vi "UHR-Fleezers Control (host) - 11.1.vi"() -> ()   [LabVIEW 2012] (continued)
            n680 = call "move to saved stage position.vi"("error in"=w1090, "Stage VISA resource name in"=w1091, "Position"="Stage Position To Establish FB", "Saved Stage Positions"=w1093) -> ("error out"=w1089:errorcluster)  [unwired: 1 out]
            n681 = local write "Stage Control Serial Error"(w1089) -> ()
          }
          frame #2 {
            n682 = call <vilib>:"Beep.vi"() -> ()  [unwired: 3 in, 9 out]
            n683 = Multiply(x="Wait (s)", y=u32 1000 ("milliseconds to wait")) -> (x*y=w1099:u32)
            n684 = property on="Trap Delta (MHz)" class="DigNum (strict)"("Val(Sgnl)"="Starting \nTrap Delta (MHz)") -> ()  [unwired: 2 in, 2 out]
            n685 = local write "Stage Moving"(FALSE ("Stage Moving")) -> ()
            n686 = Wait (ms)(milliseconds to wait=w1099) -> ()  [unwired: 1 out]
            n687 = property on="Tab Control 2" class="TabCtl (strict)"("Val(Sgnl)"=T6."Feedback on Trap Position" ("Value (Signaling)")) -> ()  [unwired: 2 in, 2 out]
            n688 = property on="Tab Control" class="TabCtl (strict)"("Val(Sgnl)"=T4."Trap Control (RF)" ("Value (Signaling)")) -> ()  [unwired: 2 in, 2 out]
          }
          frame #3 {
            n689 = property on="Set Reading to\nSetpoint" class="Bool (strict)"("Val(Sgnl)"=TRUE ("Value (Signaling)")) -> ()  [unwired: 2 in, 2 out]
            n690 = Wait (ms)(milliseconds to wait=u32 500) -> ()  [unwired: 1 out]
          }
          frame #4 {
            n691 = property on="Trap Pos. FB ON" class="Bool (strict)"("Val(Sgnl)"=TRUE ("Value (Signaling)")) -> ()  [unwired: 2 in, 2 out]
            n692 = Wait (ms)(milliseconds to wait=u32 250) -> ()  [unwired: 1 out]
          }
          frame #5 {
            n693 = case shown="False" "Trap Trig Fl." {
              frame False {
                n694 = case shown="True" "Green ON after FB ON?" {
                  selector: "Green ON after FB ON?" -> [_ w1115]
                  frame False {
                  }
                  frame True {
                    n695 = property on="Green Laser ON/Interlacing" class="Bool (strict)"("Val(Sgnl)"=w1115) -> ()  [unwired: 2 in, 2 out]
                  }
                }
              }
              frame True {
              }
            }
            n696 = case shown="True" "Remove Action Offset" {
              tunnel: TRUE ("Value (Signaling)") -> [w1112 w1113]
              frame False {
                n697 = property on="Remove Unwinding Offset" class="Bool (strict)"("Val(Sgnl)"=w1112) -> ()  [unwired: 2 in, 2 out]
              }
              frame True {
                n698 = property on="Remove Action Offset" class="Bool (strict)"("Val(Sgnl)"=w1113) -> ()  [unwired: 2 in, 2 out]
              }
            }
            n699 = Wait (ms)(milliseconds to wait=u32 250) -> ()  [unwired: 1 out]
          }
          frame #6 {
            n700 = property on="Start Saving" class="Bool (strict)"("Val(Sgnl)"=TRUE ("Value (Signaling)")) -> ()  [unwired: 2 in, 2 out]
            n701 = Wait (ms)(milliseconds to wait=u32 5000) -> ()  [unwired: 1 out]
          }
          frame #7 {
            w1119 = TRUE ("Value (Signaling)")
            n702 = property on="Rem fb disp offset" class="Bool (strict)"("Val(Sgnl)"=w1119) -> ()  [unwired: 2 in, 2 out]
            n703 = property on="Remove Offset" class="Bool (strict)"("Val(Sgnl)"=w1119) -> ()  [unwired: 2 in, 2 out]
            n704 = Wait (ms)(milliseconds to wait=u32 100) -> ()  [unwired: 1 out]
          }
          frame #8 {
            n705 = case shown="True" w1122 {
              frame False {
              }
              frame True {
                n706 = local write "Trap Trig. Fl."(TRUE ("Value (Signaling)")) -> ()
              }
            }
          }
          frame #9 {
            n707 = case shown="True" "Start dipping after?" {
              frame False {
              }
              frame True {
                n708 = flat-sequence {
                  frame #0 {
                    n709 = Multiply(x="Delay before dipping (s)", y=1000.0) -> (x*y=w1126:dbl)
                    n710 = Wait (ms)(milliseconds to wait=w1126) -> ()  [unwired: 1 out]
                  }
                  frame #1 {
                    n711 = property on="Dip for Protein" class="Bool (strict)"("Val(Sgnl)"=TRUE ("Value (Signaling)")) -> ()  [unwired: 2 in, 2 out]
                    n712 = local write "Scripts"(T1."Dipping" ("Scripts")) -> ()
                  }
                }
              }
            }
          }
        }
      }
      event "Fixed Traps Data\nScript": Value Change {
        n713 = event-data() -> ()  [unwired: 1 in, 5 out]
        n714 = flat-sequence {
          frame #0 {
            n715 = case shown="True" "Green ON" {
              frame False {
              }
              frame True {
                n716 = property on="Green Laser ON/Interlacing" class="Bool (strict)"("Val(Sgnl)"=TRUE) -> ()  [unwired: 2 in, 2 out]
              }
            }
            n717 = local write "Offset (nm)"(0.0 ("Offset (nm)")) -> ()
            n718 = property on="Sample Channel\nFlow" class="Bool (strict)"("Val(Sgnl)"=FALSE ("Value (Signaling)")) -> ()  [unwired: 2 in, 2 out]
            n719 = property on="Trap Delta (MHz)" class="DigNum (strict)"("Val(Sgnl)"="Fixed Traps Trap Delta (MHz)") -> ()  [unwired: 2 in, 2 out]
          }
          frame #1 {
            n720 = Wait (ms)(milliseconds to wait=u32 1000) -> ()  [unwired: 1 out]
          }
          frame #2 {
            n721 = local write "Start Saving"(TRUE ("Start Saving")) -> ()
          }
          frame #3 {
            n722 = local read "Bead Sep. Int. Time (s)"() -> (w1137:dbl)
            n723 = Multiply(x=w1137, y=1000.0) -> (x*y=w1139:dbl)
            n724 = Wait (ms)(milliseconds to wait=w1139) -> ()  [unwired: 1 out]
          }
          frame #4 {
            n725 = property on="Remove Offset" class="Bool (strict)"("Val(Sgnl)"=TRUE ("Value (Signaling)")) -> ()  [unwired: 2 in, 2 out]
          }
          frame #5 {
            n726 = property on="Dip for Protein" class="Bool (strict)"("Val(Sgnl)"="Start dipping after?") -> ()  [unwired: 2 in, 2 out]
          }
        }
      }
      event "Got DNA bead": Value Change {
        n727 = event-data() -> ()  [unwired: 1 in, 5 out]
        n728 = flat-sequence {
          frame #0 {
            n729 = local read "Daq spot flow on"() -> (w1144:bool)
            n730 = case shown="True" w1144 {
              frame False {
              }
              frame True {
                n731 = property on="Sample Channel\nFlow" class="Bool (strict)"("Val(Sgnl)"=TRUE ("Value (Signaling)")) -> ()  [unwired: 2 in, 2 out]
              }
            }
            n732 = property on="Got DNA bead" class="Bool"("Key Focus"=FALSE) -> ()  [unwired: 2 in, 2 out]
          }
          frame #1 {
            n733 = property on="Inject Pump 1" class="Bool (strict)"("Val(Sgnl)"=FALSE ("Value (Signaling)")) -> ()  [unwired: 2 in, 2 out]
          }
          frame #2 {
            n734 = property on="Cal/Data Acq. Spot" class="Bool (strict)"("Val(Sgnl)"=TRUE ("Value (Signaling)")) -> ()  [unwired: 2 in, 2 out]
          }
        }
      }
      event "Take Stepping Data": Value Change {
        n735 = event-data() -> ()  [unwired: 1 in, 5 out]
        n736 = local read "Save ave N"() -> (w1156:dbl)
        n737 = flat-sequence {
          tunnel: w1156 -> [w1158]
          tunnel: [w1158] -> w1151
          tunnel: [w1160] -> w1152
          tunnel: w1151 -> [w1160]
          tunnel: [w1162] -> w1153
          tunnel: w1152 -> [w1162]
          tunnel: [w1165] -> w1154
          tunnel: w1153 -> [w1165]
          tunnel: [w1167] -> w1155
          tunnel: w1154 -> [w1167]
          tunnel: [w1169] -> w1149
          tunnel: w1155 -> [w1169]
          tunnel: w1149 -> [w1172]
          tunnel: [w1172] -> w1148
          tunnel: w1148 -> [w1173]
          tunnel: [w1173] -> w1150
          tunnel: w1150 -> [w1179]
          frame #0 {
            n738 = property on="Save ave N" class="DigNum (strict)"("Val(Sgnl)"="Save ave factor") -> ()  [unwired: 2 in, 2 out]
          }
          frame #1 {
            n739 = Wait (ms)(milliseconds to wait=u32 100) -> ()  [unwired: 1 out]
          }
          frame #2 {
            n740 = local read "Offset 2 Start (MHz)"() -> (w1164:dbl)
            n741 = property on="Saved AOD Raster Scan Parameter Sets" class="Arr (strict)"("Index Values"=u32[] [2]) -> ()  [unwired: 2 in, 2 out]
            n742 = property on="Trap Delta (MHz)" class="DigNum (strict)"("Val(Sgnl)"=w1164) -> ()  [unwired: 2 in, 2 out]
          }
          frame #3 {
            n743 = property on="Load parameters" class="Bool (strict)"("Val(Sgnl)"=TRUE ("Value (Signaling)")) -> ()  [unwired: 2 in, 2 out]
          }
          frame #4 {
            n744 = Wait (ms)(milliseconds to wait=u32 100) -> ()  [unwired: 1 out]
          }
          frame #5 {
            n745 = property on="Trap Raster Scan" class="Bool (strict)"("Val(Sgnl)"=TRUE ("Value (Signaling)")) -> ()  [unwired: 2 in, 2 out]
          }
          frame #6 {
            n746 = Wait (ms)(milliseconds to wait=u32 1000) -> ()  [unwired: 1 out]
          }
          frame #7 {
            n747 = while {
              stop <- w1176 stop-if-true
              n748 = local read "Raster Scanning..."() -> (w1178:bool)
              n749 = local read "Saving..."() -> (w1177:bool)
              n750 = Not(x=w1177) -> (.not. x?=w1174:bool)
              n751 = Not(x=w1178) -> (.not. x?=w1175:bool)
              n752 = And(x=w1175, y=w1174) -> (x .and. y?=w1176:bool)
            }
          }
          frame #8 {
            n753 = property on="Save ave N" class="DigNum (strict)"("Val(Sgnl)"=w1179) -> ()  [unwired: 2 in, 2 out]
          }
        }
      }
      event "Step Size (nm)": Value Change {
        n754 = event-data() -> ()  [unwired: 1 in, 5 out]
        n755 = flat-sequence {
          frame #0 {
            n756 = property on="Saved AOD Raster Scan Parameter Sets" class="Arr (strict)"("Index Values"=u32[] [1]) -> ()  [unwired: 2 in, 2 out]
          }
          frame #1 {
            n757 = Multiply(x="N Steps", y="Step Size (nm)") -> (x*y=w1181:dbl)
            n758 = property on="Scan Speed AOD (nm/s) 2" class="DigNum (strict)"("Value"="Step Size (nm)") -> ()  [unwired: 2 in, 2 out]
            n759 = property on="Step Size AOD (nm) 2" class="DigNum (strict)"("Value"="Step Size (nm)") -> ()  [unwired: 2 in, 2 out]
            n760 = property on="Scan Range AOD (nm) 2" class="DigNum (strict)"("Value"=w1181) -> ()  [unwired: 2 in, 2 out]
          }
        }
      }
      event "Take Detection Laser\nImage": Value Change {
        n761 = event-data() -> ()  [unwired: 1 in, 5 out]
        n762 = flat-sequence {
          tunnel: [w1209] -> w1199
          tunnel: [w1208] -> w1192
          tunnel: [w1207] -> w1184
          tunnel: [w1212] -> w1200
          tunnel: w1199 -> [w1212]
          tunnel: [w1211] -> w1193
          tunnel: w1192 -> [w1211]
          tunnel: [w1210] -> w1185
          tunnel: w1184 -> [w1210]
          tunnel: [w1216] -> w1201
          tunnel: w1200 -> [w1216]
          tunnel: [w1215] -> w1194
          tunnel: w1193 -> [w1215]
          tunnel: [w1214] -> w1186
          tunnel: w1185 -> [w1214]
          tunnel: [w1222] -> w1202
          tunnel: w1201 -> [w1222]
          tunnel: [w1221] -> w1195
          tunnel: w1194 -> [w1221]
          tunnel: [w1220] -> w1187
          tunnel: w1186 -> [w1220]
          tunnel: [w1226] -> w1203
          tunnel: w1202 -> [w1226]
          tunnel: [w1225] -> w1196
          tunnel: w1195 -> [w1225]
          tunnel: [w1224] -> w1188
          tunnel: w1187 -> [w1224]
          tunnel: [w1230] -> w1204
          tunnel: w1203 -> [w1230]
          tunnel: [w1229] -> w1197
          tunnel: w1196 -> [w1229]
          tunnel: [w1228] -> w1189
          tunnel: w1188 -> [w1228]
          tunnel: [w1234] -> w1205
          tunnel: w1204 -> [w1234]
          tunnel: [w1233] -> w1198
          tunnel: w1197 -> [w1233]
          tunnel: [w1232] -> w1190
          tunnel: w1189 -> [w1232]
          tunnel: w1205 -> [w1240]
          tunnel: w1198 -> [w1239]
          tunnel: [w1237] -> w1191
          tunnel: w1190 -> [w1237]
          tunnel: w1191 -> [w1241]
          frame #0 {
            n763 = local read "Green Laser ON/Interlacing"() -> (w1209:bool)
            n764 = local read "Green laser mode"() -> (w1208:enum32{"Laser ON", "Laser OFF", "Interlace"})
            n765 = local read "Green FB On/Off"() -> (w1207:bool)
          }
          frame #1 {
            n766 = property on="Green FB On/Off" class="Bool (strict)"("Val(Sgnl)"=FALSE ("Value (Signaling)")) -> ()  [unwired: 2 in, 2 out]
          }
          frame #2 {
            n767 = property on="Green Laser ON/Interlacing" class="Bool (strict)"("Val(Sgnl)"=TRUE ("Value (Signaling)")) -> ()  [unwired: 2 in, 2 out]
            n768 = property on="Flip Green Filter" class="Bool (strict)"("Val(Sgnl)"=TRUE ("Value (Signaling)")) -> ()  [unwired: 2 in, 2 out]
            n769 = property on="Green laser mode" class="RadioBtnsControl (strict)"("Val(Sgnl)"=enum32{"Laser ON", "Laser OFF", "Interlace"}."Laser ON" ("Value (Signaling)")) -> ()  [unwired: 2 in, 2 out]
          }
          frame #3 {
            n770 = Wait (ms)(milliseconds to wait=u32 500) -> ()  [unwired: 1 out]
          }
          frame #4 {
            n771 = property on="Confocal Image" class="Bool (strict)"("Val(Sgnl)"=TRUE ("Value (Signaling)")) -> ()  [unwired: 2 in, 2 out]
          }
          frame #5 {
            n772 = Wait (ms)(milliseconds to wait=u32 2000) -> ()  [unwired: 1 out]
          }
          frame #6 {
            n773 = while {
              stop <- w1235 stop-if-true
              n774 = local read "Saving..."() -> (w1236:bool)
              n775 = Not(x=w1236) -> (.not. x?=w1235:bool)
            }
          }
          frame #7 {
            n776 = property on="Flip Green Filter" class="Bool (strict)"("Val(Sgnl)"=TRUE ("Value (Signaling)")) -> ()  [unwired: 2 in, 2 out]
            n777 = property on="Green Laser ON/Interlacing" class="Bool (strict)"("Val(Sgnl)"=w1240) -> ()  [unwired: 2 in, 2 out]
            n778 = property on="Green laser mode" class="RadioBtnsControl (strict)"("Val(Sgnl)"=w1239) -> ()  [unwired: 2 in, 2 out]
          }
          frame #8 {
            n779 = property on="Green FB On/Off" class="Bool (strict)"("Val(Sgnl)"=w1241) -> ()  [unwired: 2 in, 2 out]
          }
        }
      }
      event "Stop All": Value Change {
        n780 = event-data() -> ()  [unwired: 1 in, 5 out]
        n781 = local read "Stop All"() -> (w1242:bool)
      }
    }
    n782 = node-c288() -> ()  [unwired: 1 in, 1 out]
  }
  n783 = node-c288(3 ("Processor")) -> (w95:T21)  [unwired: 3 out]
  n784 = flat-sequence "Video" {
    tunnel: [w1251] -> w85
    tunnel: w85 -> [w1292]
    frame #0 {
      n785 = while {
        stop <- w1244 continue-if-true
        n786 = call "Close Video Capture.vi"() -> ("error code OUT"=w1246:i32)
        n787 = Equal?(x=w1246, y=0) -> (x = y?=w1244:bool)
      }
      n788 = local write "Stop All"(FALSE ("Stop All")) -> ()
    }
    frame #1 {
      n789 = call "DMR_Init.vi"() -> ()  [unwired: 3 out]
    }
    frame #2 {
      # "Setting the destination format to Mono8 makes sure that the image can be displayed in the intensity plot."
      n790 = call "DMR_GetDevice.vi"("search string IN"="DE019116701") -> ("device handle OUT"=w1269:i32)  [unwired: 4 in, 2 out]
      n791 = call "DMR_OpenDevice.vi"("device handle IN"=w1269) -> ("driver handle OUT"=w1252:i32)  [unwired: 4 out]
      n792 = call "DMR_FindList.vi"("flags IN"=u32 0 ("flags"), "list name IN"="" ("String"), "list type IN"=T26."camera descriptions", "driver handle IN"=w1252) -> ("list handle OUT"=w1255:i32)  [unwired: 2 out]
      n793 = call "DMR_FindList.vi"("flags IN"=u32 0 ("flags"), "list name IN"="Base", "list type IN"=T26."setting", "driver handle IN"=w1252) -> ("list handle OUT"=w1253:i32)  [unwired: 2 out]
      n794 = call "OBJ_GetHandle.vi"("object name IN"="VideoStandard", "list handle IN"=w1255) -> ("object handle OUT"=w1249:i32)  [unwired: 3 out]
      n795 = call "OBJ_GetHandle.vi"("object name IN"="PixelFormat", "list handle IN"=w1253) -> ("object handle OUT"=w1263:i32)  [unwired: 3 out]
      n796 = call "OBJ_SetS.vi"("value index IN"=0, "value IN"="NTSC M", "object handle IN"=w1249) -> ()  [unwired: 2 out]
      n797 = call "OBJ_SetS.vi"("value index IN"=0, "value IN"="Mono8" ("value"), "object handle IN"=w1263) -> ()  [unwired: 2 out]
      n798 = call "OBJ_GetHandle.vi"("object name IN"="VideoChannel", "list handle IN"=w1253) -> ("object handle OUT"=w1259:i32)  [unwired: 3 out]
      n799 = while {
        tunnel: [w1274] -> w1251
        tunnel: w1252 -> [w1271]
        stop <- w1272 continue-if-true
        n800 = call "DMR_ImageRequestSingle.vi"("request control IN"=0, "driver handle IN"=w1271) -> ("error code OUT"=w1273:i32, "driver handle OUT"=w1274:i32)  [unwired: 2 out]
        n801 = Equal To 0?(x=w1273) -> (x = 0?=w1272:bool)
      }
      n802 = call "OBJ_SetI.vi"("value index IN"=0, "value IN"=3 ("Video channel"), "object handle IN"=w1259) -> ()  [unwired: 2 out]
    }
    frame #3 {
      w1280 = T17 0 items=["Grayscale (U8)", "Grayscale (I16)", "Grayscale (SGL)", "Complex (CSG)", "RGB (U32)", "HSL (U32)", "RGB (U64)"] ("Image Type")
      w1288 = T17 0 items=["Grayscale (U8)", "Grayscale (I16)", "Grayscale (SGL)", "Complex (CSG)", "RGB (U32)", "HSL (U32)", "RGB (U64)"] ("Image Type")
      n803 = for "Create Greyscale map" {
        N: 256 -> [_]
        tunnel: [w1294] -> w1277 mode=indexing
        workers-P: _ -> [_]
        i -> [w1297]
        n804 = To Unsigned Byte Integer(number=w1297) -> (unsigned 8bit integer=w1293:u8)
        n805 = Join Numbers(hi=w1293, lo=w1293) -> ((hi.lo)=w1296:u16)
        n806 = Join Numbers(hi=w1293, lo=w1293) -> ((hi.lo)=w1295:u16)
        n807 = Join Numbers(hi=w1296, lo=w1295) -> ((hi.lo)=w1294:u32)
      }
      n808 = call "IMAQ Create"("Image Name"="Scaled video", "Image Type"=w1280) -> ("New Image"=w1279:T2)  [unwired: 2 in, 2 out]
      n809 = call "IMAQ Create"("Image Name"="Main video", "Image Type"=w1288) -> ("New Image"=w1289:T2)  [unwired: 2 in, 2 out]
      n810 = node-c288(0 ("Processor")) -> (w1287:T21)  [unwired: 3 out]
      n811 = Initialize Array(u32 0 ("Window Number (0...15)"), 480 ("dimension size"), 640 ("dimension size")) -> (w1282:u32[][])
      n812 = timed-loop {
        tunnel: w1292 -> [w1314]
        tunnel: [w1313] -> w1291
        tunnel: w1289 -> [w1312]
        timing: w1287 -> [_]
        timing-out: [_] -> w1286
        tunnel: w1282 -> [w1301]
        tunnel: w1279 -> [w1299]
        tunnel: w1277 -> [w1298]
        stop <- w1300 stop-if-true
        # "This block performs the \nactual image capture."
        n813 = node-c288() -> ()  [unwired: 2 out]
        n814 = local read "Stop All"() -> (w1300:bool)
        n815 = Reciprocal(x="Video Capture Rate (Hz)") -> (1/x=w1304:dbl)
        n816 = Multiply(x=w1304, y=1000.0) -> (x*y=w1302:dbl)
        n817 = call "DMR_ImageRequestWaitFor.vi"("queue number IN"=0, "timeout(ms) IN"=500, "driver handle IN"=w1314) -> ("error code OUT"=w1318:i32, "request number OUT"=w1315:i32, "driver handle OUT"=w1316:i32)
        n818 = feedback #1(T27 refnum ("Avi Refnum")) -> (w1306:T27)
        n819 = case shown="True" "New Video File" {
          tunnel: [T27 refnum ("Avi Refnum") w1335] -> w1308
          tunnel: [FALSE TRUE] -> w1309
          tunnel: w1306 -> [_ w1331]
          frame False {
          }
          frame True {
            n820 = call "Create new save file.vi"("Ext"=".avi" ("string"), "Index In"="Video Index") -> ("Path Out"=w1327:path, "Index Out"=w1328:dbl)  [unwired: 1 in]
            "Path Out" <- w1327
            n821 = Not Equal?(x=w1331, y=T27 refnum ("Avi Refnum")) -> (x != y?=w1332:bool)
            n822 = Increment(x=w1328) -> (x+1=w1337:dbl)
            n823 = case shown="True" w1332 {
              tunnel: w1331 -> [_ w1338]
              frame False {
              }
              frame True {
                n824 = call "IMAQ AVI Close"("Avi Refnum"=w1338) -> ()  [unwired: 1 in, 10 out]
              }
            }
            n825 = local write "Video Index"(w1337) -> ()
            n826 = call "IMAQ AVI Create"("Frames Per Second"=u32 30, "AVI Path"=w1327) -> ("Avi Refnum"=w1335:T27)  [unwired: 5 in, 4 out]
          }
        }
        n827 = Equal To 0?(x=w1318) -> (x = 0?=w1317:bool)
        n828 = Select(t=w1308, s=w1309, f=w1306) -> (s? t:f=w1307:T27)
        n829 = feedback-in #1(w1307) -> ()
        n830 = case shown="True" w1317 {
          tunnel: w1316 -> [w1339 w1364]
          tunnel: w1315 -> [_ w1363]
          tunnel: [w1339 w1360] -> w1313
          tunnel: w1312 -> [_ w1344]
          tunnel: w1301 -> [_ w1348]
          tunnel: w1307 -> [_ w1346]
          tunnel: w1299 -> [_ w1341]
          tunnel: w1298 -> [_ w1340]
          frame False {
          }
          frame True {
            w1354 = u32 0 ("X-offset IN")
            n831 = call "DMR_GetImageRequestBufferData.vi"("driver handle IN"=w1364, "request number IN"=w1363) -> ("width OUT"=w1353:i32, "height OUT"=w1352:i32, "driver handle OUT"=w1359:i32, "request number OUT"=w1358:i32, "bytes per pixel OUT"=w1355:i32)  [unwired: 13 out]
            n832 = call "DMR_GetImageRequestBufferImageData.vi"("driver handle IN"=w1359, "request number IN"=w1358, "bytes per pixel IN"=w1355, "X-offset IN"=w1354, "Y-offset IN"=w1354, "height IN"=w1352, "width IN"=w1353) -> ("driver handle OUT"=w1357:u32, "request number OUT"=w1356:u32, "image OUT"=w1349:u32[][])  [unwired: 10 out]
            n833 = call "DMR_ImageRequestUnlock.vi"("request number IN"=w1356, "driver handle IN"=w1357) -> ("driver handle OUT"=w1362:i32)  [unwired: 1 in, 2 out]
            n834 = case shown="True" "Averaging" {
              tunnel: w1349 -> [w1400 w1405]
              tunnel: [w1400 w1404] -> w1345
              tunnel: w1348 -> [_ w1402]
              frame False {
              }
              frame True {
                (unwired) 1
                w1410 = 1
                n835 = feedback #2(w1402) -> (w1401:u32[][])
                n836 = Add(x=w1405, y=w1401) -> (x+y=w1406:u32[][])
                n837 = Select(t=w1402, s="Reset Averaging", f=w1406) -> (s? t:f=w1408:u32[][])
                n838 = feedback-in #2(w1408) -> ()
                n839 = feedback #3(w1410) -> (w1403:i32)
                n840 = Divide(x=w1406, y=w1403) -> (x/y=w1407:dbl[][])
                n841 = Increment(x=w1403) -> (x+1=w1411:i32)
                n842 = To Unsigned Long Integer(number=w1407) -> (unsigned 32bit integer=w1404:u32[][])
                n843 = Select(t=w1410, s="Reset Averaging", f=w1411) -> (s? t:f=w1409:i32)
                n844 = feedback-in #3(w1409) -> ()
              }
            }
            n845 = call "DMR_ImageRequestSingle.vi"("request control IN"=0, "driver handle IN"=w1362) -> ("driver handle OUT"=w1360:i32)  [unwired: 3 out]
            n846 = disable-structure shown="Disabled" {
              disable-tunnel: w1345 -> [w1377 _]
              disable-tunnel: w1341 -> [w1376 _]
              frame Disabled {
                n847 = To Double Precision Float(number=w1377) -> (double precision float=w1375:dbl[][])
                n848 = In Range and Coerce(upper limit="Intensity Upper", x=w1375, lower limit="Intensity Lower") -> (coerced(x)=w1374:dbl[][])  [unwired: 1 out]
                n849 = Subtract(x="Intensity Upper", y="Intensity Lower") -> (x-y=w1371:dbl)
                n850 = Subtract(x=w1374, y="Intensity Lower") -> (x-y=w1372:dbl[][])
                n851 = Divide(x=w1372, y=w1371) -> (x/y=w1373:dbl[][])
                n852 = Multiply(x=255.0, y=w1373) -> (x*y=w1369:dbl[][])
                n853 = To Unsigned Byte Integer(number=w1369) -> (unsigned 8bit integer=w1378:u8[][])
                n854 = call "IMAQ ArrayToImage"("Image Pixels (U8)"=w1378, "Image"=w1376) -> ("Image Out"=w1365:T2)  [unwired: 4 in, 5 out]
                n855 = First Call?() -> (First Call?: T/F=w1366:bool)
                n856 = case shown="True" w1366 {
                  tunnel: w1365 -> [w1379 w1390]
                  frame False {
                    n857 = flat-sequence {
                      tunnel: w1379 -> [w1385]
                      frame #0 {
                        w1382 = FALSE ("Get/Set Status? (Set)")
                        w1381 = 0 ("Window Number (0...15)")
                        n858 = call "IMAQ WindSize"("Get/Set Status? (Set)"=w1382, "Window Number"=w1381) -> ("Width & Height out"=→"Window Size":cluster{"Width":i32, "Height":i32})  [unwired: 4 in, 2 out]
                        n859 = call "IMAQ WindMove"("Window Number (0...15)"=w1381, "Get/Set Status? (Set)"=w1382) -> ("Coordinates (screen)"=→"Window Position":cluster{"X Position":i32, "Y Position":i32})  [unwired: 3 in, 1 out]
                        n860 = call "IMAQ WindDraw"("Resize to Image Size? (Y)"=FALSE, "Window Number (0...15)"=w1381, "Image"=w1385) -> ()  [unwired: 7 in, 2 out]
                      }
                      frame #1 {
                        n861 = call "IMAQ WindZoom 2"("Center Point"="Center Point", "Zoom to Fit? (False)"=FALSE, "Zoom Factor"="Zoom Factor") -> ()  [unwired: 5 in, 4 out]
                      }
                    }
                  }
                  frame True {
                    n862 = flat-sequence {
                      tunnel: w1390 -> [w1393]
                      tunnel: [w1391] -> w1389
                      tunnel: w1389 -> [w1395]
                      frame #0 {
                        w1392 = TRUE ("Resize to Image Size? (Y)")
                        w1391 = 0 ("Window Number (0...15)")
                        n863 = call "IMAQ WindNonTearing"("Window Number"=w1391, "NonTearing? (True)"=w1392) -> ()  [unwired: 8 in, 2 out]
                        n864 = call "IMAQ WindDraw"("Resize to Image Size? (Y)"=w1392, "Window Number (0...15)"=w1391, "Image"=w1393) -> ()  [unwired: 7 in, 2 out]
                      }
                      frame #1 {
                        n865 = call "IMAQ WindSize"("Scrollbars? (N)"=FALSE, "Width & Height"="Initial Window Size", "Window Number"=w1395) -> ()  [unwired: 3 in, 3 out]
                        n866 = call "IMAQ WindMove"("Window Number (0...15)"=w1395, "Coordinates (screen)"="Initial Window Position") -> ()  [unwired: 3 in, 2 out]
                      }
                    }
                  }
                }
              }
              frame Enabled {
              }
            }
            n867 = To Unsigned Byte Integer(number=w1345) -> (unsigned 8bit integer=w1343:u8[][])
            n868 = call "IMAQ ArrayToImage"("Image Pixels (U8)"=w1343, "Image"=w1344) -> ("Image Out"=w1342:T2)  [unwired: 4 in, 5 out]
            "Primary Video Display" <- w1342
            n869 = case shown="True" "Save Video" {
              tunnel: w1346 -> [_ w1399]
              tunnel: w1342 -> [_ w1398]
              frame False {
              }
              frame True {
                n870 = call "IMAQ AVI Write Frame"("Image"=w1398, "Avi Refnum"=w1399) -> ()  [unwired: 2 in, 8 out]
              }
            }
            n871 = case shown="True" "Save Image" {
              tunnel: w1343 -> [_ w1414]
              tunnel: w1340 -> [_ w1413]
              frame False {
              }
              frame True {
                n872 = call <vilib>:"Flatten Pixmap.vi"("colors"=w1413, "8-bit pixmap"=w1414) -> ("image data"=w1420:T28)  [unwired: 4 in, 5 out]
                n873 = call "Create new save file.vi"("Insert"="video_frame_" ("string"), "Ext"=".bmp" ("string"), "Index In"="Image Index") -> ("Path Out"=w1416:path, "Index Out"=w1421:dbl)
                n874 = Increment(x=w1421) -> (x+1=w1415:dbl)
                n875 = local write "Image Index"(w1415) -> ()
                n876 = call <vilib>:"Write BMP File.vi"("image data"=w1420, "path to BMP file"=w1416) -> ()  [unwired: 1 in, 9 out]
              }
            }
          }
        }
        n877 = node-c288(w1302) -> ()  [unwired: 1 out]
      }
      n878 = node-c288(w1286) -> ()  [unwired: 1 out]
      n879 = call "DMR_CloseDevice.vi"("driver handle IN"=w1291) -> ()  [unwired: 1 in, 4 out]
    }
    frame #4 {
      n880 = call "DMR_Close.vi"() -> ()  [unwired: 1 out]
    }
  }
  n881 = timed-loop "Acquire Data" {
    tunnel: w6 -> [w1720]
    tunnel: w55 -> [w1719]
    tunnel: [w1749] -> w275
    tunnel: [w1744] -> w273
    timing: w180 -> [_]
    timing-out: [_] -> w179
    tunnel: w74 -> [w1557]
    stop <- "Stop All" stop-if-true
    w1472 = "Initialize"
    w1542 = "NI_ChannelName" ("name")
    n882 = node-c288() -> ()  [unwired: 2 out]
    n883 = First Call?() -> (First Call?: T/F=w1507:bool)
    n884 = Or(x="Reset", y=w1507) -> (x .or. y?=w1508:bool)
    n885 = local read "Flushing P1"() -> (w1427:bool)
    n886 = case "Reset data stream" shown="True" w1508 {
      tunnel: w1720 -> [w2725 w2733]
      tunnel: w1719 -> [w2724 w2732]
      tunnel: [w2725 w2727] -> w1715
      tunnel: [w2724 w2726] -> w1714
      frame False {
      }
      frame True {
        w2730 = TRUE ("AI to FIFO")
        n887 = local write "Overflow (data lost)"(FALSE ("Overflow (data lost)")) -> ()
        n888 = call "reset FPGA DMA.vi"("error in"=w2732, "FPGA VI Reference In"=w2733) -> ("error out"=w2728:errorcluster, "FPGA VI Reference Out"=w2729:T19)
        n889 = xnode "Read/Write Control"("FPGA VI Reference In"=w2729, "error in"=w2728, "AI to FIFO"=w2730, "APD to FIFO"=w2730) -> ("FPGA VI Reference Out"=w2727:T19, "error out"=w2726:errorcluster)
      }
    }
    n890 = case shown="True" w1427 {
      frame False {
      }
      frame True {
        n891 = local read "Flush rate (uL/m) P1"() -> (w1766:dbl)
        n892 = local read "HP1 Flush Time (s)"() -> (w1775:dbl)
        n893 = local read "DMA Update Period (s)"() -> (w1769:dbl)
        n894 = Divide(x=w1766, y=60.0) -> (x/y=w1767:dbl)
        n895 = Divide(x=w1775, y=w1769) -> (x/y=w1764:dbl)
        n896 = feedback #4(0) -> (w1773:i32)
        n897 = Increment(x=w1773) -> (x+1=w1763:i32)
        n898 = Greater?(x=w1763, y=w1764) -> (0:w1772:bool)
        n899 = Compound Arithmetic op=MULTIPLY(w1769, w1763, w1767) -> (→"P1 Flush Volume (uL)":dbl)
        n900 = Divide(x=w1763, y=w1764) -> (x/y=→"P1 Flushing Bar":dbl)
        n901 = case shown="True" w1772 {
          tunnel: w1763 -> [w1776 _]
          tunnel: [w1776 0] -> w1771
          frame False {
          }
          frame True {
            w1777 = FALSE ("Flushing P1")
            n902 = local write "Inject Pump 1"(w1777) -> ()
            n903 = local write "Flushing P1"(w1777) -> ()
            n904 = property on="Clear Volume P1" class="Bool (strict)"("Val(Sgnl)"=TRUE ("Value (Signaling)")) -> ()  [unwired: 2 in, 2 out]
          }
        }
        n905 = feedback-in #4(w1771) -> ()
      }
    }
    n906 = Or(x="Start AOD Scan", y="Trap Raster Scan") -> (x .or. y?=w1665:bool)
    n907 = case "Start AOM raster scan" shown="True" w1665 {
      tunnel: w1715 -> [w2575 w2585]
      tunnel: w1714 -> [w2574 w2584]
      tunnel: [w2575 w2578] -> w1713
      tunnel: [w2574 w2577] -> w1712
      frame False {
      }
      frame True {
        n908 = case shown="True" "Restart DMA? (AOD)" {
          tunnel: [w2623 w2625] -> w2579
          tunnel: [w2622 w2624] -> w2580
          tunnel: w2585 -> [w2623 w2627]
          tunnel: w2584 -> [w2622 w2626]
          frame False {
          }
          frame True {
            n909 = local write "Overflow (data lost)"(FALSE ("Overflow (data lost)")) -> ()
            n910 = call "reset FPGA DMA.vi"("error in"=w2626, "FPGA VI Reference In"=w2627) -> ("error out"=w2624:errorcluster, "FPGA VI Reference Out"=w2625:T19)
          }
        }
        n911 = local write "Trap Raster Scan"(FALSE ("Trap Raster Scan")) -> ()
        n912 = case shown="True" "Move MCL Also?" {
          tunnel: w2580 -> [w2588 w2617]
          tunnel: w2579 -> [w2589 w2618]
          tunnel: [w2587 w2621] -> w2578
          tunnel: [w2586 w2620] -> w2577
          frame False {
            w2590 = TRUE ("AI to FIFO")
            n913 = xnode "Read/Write Control"("FPGA VI Reference In"=w2589, "error in"=w2588, "AI to FIFO"=w2590, "APD to FIFO"=w2590, "Start scan"=w2590) -> ("FPGA VI Reference Out"=w2587:T19, "error out"=w2586:errorcluster)
          }
          frame True {
            w2614 = FALSE ("1D or 2D Scan?")
            w2619 = TRUE ("AI to FIFO")
            # "Count for MCL loop"
            # "N total cycles"
            # "N steps"
            # "V_int"
            n914 = local read "Scan Range (nm)"() -> (w2596:dbl)
            n915 = local read "Number of F/B Scans (AOD)"() -> (w2613:u16)
            n916 = Sign(1:w2596) -> (0:w2595:dbl)
            n917 = Compound Arithmetic op=MULTIPLY(w2596, "MCL Step Position Ratio", "MCL/AOM Scale Tweak") -> (w2600:dbl)
            n918 = Negate(x=w2595) -> (-x=w2592:dbl)
            n919 = Multiply(x=w2592, y="MCL Step Increment (V_int)") -> (x*y=w2594:dbl)
            n920 = Divide(x=w2600, y="MCL X Cal (nm/V)") -> (x/y=w2606:dbl)
            n921 = Multiply(x=32767.0 ("y"), y=w2606) -> (x*y=w2612:dbl)
            n922 = local read "Total Counts (ticks)"() -> (w2597:u32)
            n923 = local read "Cycles/step (AOD)"() -> (w2608:u64)
            n924 = local read "Scan steps (AOD)"() -> (w2609:u64)
            n925 = Divide(x=w2612, y=10.0) -> (x/y=w2605:dbl)
            n926 = Divide(x=w2605, y="MCL Step Increment (V_int)") -> (x/y=w2603:dbl)
            n927 = Absolute Value(x=w2603) -> (abs(x)=w2591:dbl)
            n928 = Compound Arithmetic op=MULTIPLY(w2609, w2608, w2597) -> (w2604:u64)
            n929 = local write "wait to reset values"(w2619) -> ()
            n930 = local write "MCL Scanning"(w2619) -> ()
            n931 = Divide(x=w2604, y=w2591) -> (x/y=w2601:dbl)
            "MCL Count" <- w2601
            n932 = xnode "Read/Write Control"("FPGA VI Reference In"=w2618, "error in"=w2617, "Scan steps (MCL)"=w2591, "Number of scans (MCL)"=w2613, "Cycles per step (MCL)"=u64 1, "Scan freq.  increment (MCL)"=w2594, "1D or 2D Scan?"=w2614, "MCL Scan Axis"=w2614, "Cont. Scan (MCL)"=w2614, "MCL count"=w2601) -> ("FPGA VI Reference Out"=w2616:T19, "error out"=w2615:errorcluster)
            n933 = xnode "Read/Write Control"("FPGA VI Reference In"=w2616, "error in"=w2615, "AI to FIFO"=w2619, "APD to FIFO"=w2619, "Start scan"=w2619, "Start scan (MCL)"=w2619) -> ("FPGA VI Reference Out"=w2621:T19, "error out"=w2620:errorcluster)
          }
        }
        "Raster Scanning..." <- TRUE ("Scanning...")
      }
    }
    n934 = local read "Flushing P3"() -> (w1428:bool)
    n935 = case "Keep track of when Harvard Pump 3 is done flushing" shown="True" w1428 {
      frame False {
      }
      frame True {
        n936 = local read "Flush rate (uL/m) P3"() -> (w1783:dbl)
        n937 = local read "DMA Update Period (s)"() -> (w1785:dbl)
        n938 = local read "HP3 Flush Time (s)"() -> (w1792:dbl)
        n939 = Divide(x=w1783, y=60.0) -> (x/y=w1781:dbl)
        n940 = feedback #5(0) -> (w1790:i32)
        n941 = Increment(x=w1790) -> (x+1=w1784:i32)
        n942 = Divide(x=w1792, y=w1785) -> (x/y=w1786:dbl)
        n943 = Greater?(x=w1784, y=w1786) -> (0:w1789:bool)
        n944 = Compound Arithmetic op=MULTIPLY(w1785, w1784, w1781) -> (→"P3 Flush Volume (uL)":dbl)
        n945 = case shown="True" w1789 {
          tunnel: w1784 -> [w1793 _]
          tunnel: [w1793 0] -> w1788
          frame False {
          }
          frame True {
            w1794 = FALSE ("Flushing P3")
            n946 = local write "Inject Pump 3"(w1794) -> ()
            n947 = local write "Flushing P3"(w1794) -> ()
            n948 = property on="Clear Volume P3" class="Bool (strict)"("Val(Sgnl)"=TRUE ("Value (Signaling)")) -> ()  [unwired: 2 in, 2 out]
          }
        }
        n949 = feedback-in #5(w1788) -> ()
        n950 = Divide(x=w1784, y=w1786) -> (x/y=→"P3 Flushing Bar":dbl)
      }
    }
    n951 = And(x="Save scans", y=w1665) -> (x .and. y?=w1711:bool)
    n952 = Compound Arithmetic op=OR("Start MCL Scan", "Confocal Image", "Confocal Linescan") -> (w1663:bool)
    n953 = And(x="Save Data (MCL)", y=w1663) -> (x .and. y?=w1710:bool)
    n954 = case "Start MCL raster scan" shown="True" w1663 {
      tunnel: w1713 -> [w2192 w2208]
      tunnel: w1712 -> [w2191 w2207]
      tunnel: [w2192 w2203] -> w1555
      tunnel: [w2191 w2202] -> w1554
      tunnel: [FALSE w2201] -> w1696
      tunnel: "Start MCL Scan" -> [_ w2196]
      tunnel: "Confocal Image" -> [_ w2195]
      tunnel: "Confocal Linescan" -> [_ _]
      frame False {
      }
      frame True {
        w2201 = TRUE
        n955 = case shown="True" "Restart DMA? (MCL)" {
          tunnel: [w2253 w2255] -> w2206
          tunnel: [w2252 w2254] -> w2205
          tunnel: w2208 -> [w2253 w2258]
          tunnel: w2207 -> [w2252 w2257]
          frame False {
          }
          frame True {
            n956 = call "reset FPGA DMA.vi"("error in"=w2257, "FPGA VI Reference In"=w2258) -> ("error out"=w2254:errorcluster, "FPGA VI Reference Out"=w2255:T19)
            n957 = local write "Overflow (data lost)"(FALSE ("Overflow (data lost)")) -> ()
          }
        }
        n958 = case shown="False" w2196 {
          selector: w2196 -> [_ w2212]
          tunnel: w2195 -> [w2211 _]
          tunnel: [w2211 w2212] -> w2194
          frame False {
            n959 = property on="2D or 1D Scan" class="Bool (strict)"("Val(Sgnl)"=w2211) -> ()  [unwired: 2 in, 2 out]
            n960 = property on="Confocal Image" class="Bool (strict)"("Value"=FALSE ("Start Confocal Map")) -> ()  [unwired: 2 in, 2 out]
          }
          frame True {
          }
        }
        n961 = local write "MCL Scanning"(w2201) -> ()
        n962 = local read "AO1"() -> (w2198:dbl)
        n963 = local read "AO2"() -> (w2197:dbl)
        n964 = case shown="True" "Center Scan" {
          tunnel: w2206 -> [w2219 w2251]
          tunnel: w2205 -> [w2218 w2250]
          tunnel: [w2217 w2249] -> w2203
          tunnel: [w2216 w2248] -> w2202
          tunnel: [w2214 w2235] -> w2200
          tunnel: [w2213 w2234] -> w2199
          tunnel: w2198 -> [w2214 w2240]
          tunnel: w2197 -> [w2213 w2243]
          tunnel: w2194 -> [_ _]
          frame False {
            w2215 = TRUE ("AI to FIFO")
            n965 = xnode "Read/Write Control"("FPGA VI Reference In"=w2219, "error in"=w2218, "AI to FIFO"=w2215, "APD to FIFO"=w2215, "Start scan (MCL)"=w2215) -> ("FPGA VI Reference Out"=w2217:T19, "error out"=w2216:errorcluster)
          }
          frame True {
            w2247 = TRUE ("AI to FIFO")
            n966 = local read "Scan steps (MCL)"() -> (w2226:u64)
            n967 = local read "Scan lines (y)"() -> (w2222:u64)
            n968 = local read "Fast Scan Dir"() -> (w2233:bool)
            n969 = local read "Actual MCL Inc (V)"() -> (w2223:dbl)
            n970 = Decrement(x=w2222) -> (x-1=w2221:u64)
            n971 = Decrement(x=w2226) -> (x-1=w2225:u64)
            n972 = Multiply(x=w2223, y=w2221) -> (x*y=w2220:dbl)
            n973 = Divide(x=w2220, y=2.0) -> (x/y=w2230:dbl)
            n974 = Multiply(x=w2223, y=w2225) -> (x*y=w2224:dbl)
            n975 = Divide(x=w2224, y=2.0) -> (x/y=w2229:dbl)
            n976 = Select(t=w2229, s=w2233, f=w2230) -> (s? t:f=w2228:dbl)
            n977 = Select(t=w2230, s=w2233, f=w2229) -> (s? t:f=w2232:dbl)
            n978 = Subtract(x=w2240, y=w2232) -> (x-y=w2231:dbl)
            n979 = Subtract(x=w2243, y=w2228) -> (x-y=w2227:dbl)
            n980 = local read "2D or 1D Scan"() -> (w2245:bool)
            n981 = Not(x=w2233) -> (.not. x?=w2239:bool)
            n982 = Not(x=w2245) -> (.not. x?=w2241:bool)
            n983 = And(x=w2233, y=w2241) -> (x .and. y?=w2242:bool)
            n984 = And(x=w2241, y=w2239) -> (x .and. y?=w2244:bool)
            n985 = Select(t=w2243, s=w2244, f=w2227) -> (s? t:f=w2234:dbl)
            n986 = Select(t=w2240, s=w2242, f=w2231) -> (s? t:f=w2235:dbl)
            n987 = call "Volt to I16.vi"("Voltage In"=w2235) -> ("I16 Voltage Out"=w2238:i16)
            n988 = call "Volt to I16.vi"("Voltage In"=w2234) -> ("I16 Voltage Out"=w2237:i16)
            n989 = xnode "Read/Write Control"("FPGA VI Reference In"=w2251, "error in"=w2250, "AI to FIFO"=w2247, "APD to FIFO"=w2247, "Start scan (MCL)"=w2247, "AO1"=w2238, "AO2"=w2237) -> ("FPGA VI Reference Out"=w2249:T19, "error out"=w2248:errorcluster)
          }
        }
        "Initial Y" <- w2200
        "Initial X" <- w2199
        n990 = local write "Tab Control 6"(T3."Imaging" ("Tab Control 6")) -> ()
        "wait to reset values" <- w2201
      }
    }
    n991 = local read "Trap Pos Elements/DMA read"() -> (w1551:u32)
    n992 = local read "Trap AI Elements/DMA read"() -> (w1626:u32)
    n993 = local read "APD Elements/DMA read"() -> (w1592:u32)
    n994 = xnode "Get APD Data"("FPGA VI Reference In"=w1555, "error in"=w1554, "Number of Elements"=w1592, "Timeout (ms)"=-1) -> ("Data"=w1591:void[], "Elements Remaining"=→"APD FIFO Elements Remaining")  [unwired: 2 out]
    n995 = xnode "Invoke Method"("FPGA VI Reference In"=w1555, "error in"=w1554, "Number of Elements"=w1551, "Timeout (ms)"=-1) -> ("Data"=w1514:void[], "Elements Remaining"=→"Trap Pos FIFO El Remaining")  [unwired: 2 out]
    n996 = xnode "Get Trap Data"("FPGA VI Reference In"=w1555, "error in"=w1554, "Number of Elements"=w1626, "Timeout (ms)"=-1 ("Timeout")) -> ("FPGA VI Reference Out"=w1449:T19, "error out"=w1448:errorcluster, "Data"=w1515:void[], "Elements Remaining"=w1757)
    "FIFO El. Rem." <- w1757
    n997 = local read "Trap AI FIFO Depth"() -> (w1759:u32)
    n998 = Subtract(x=w1759, y=w1626) -> (x-y=w1758:u32)
    n999 = Decimate 1D Array(w1514) -> (w1511:void[], w1513:void[], w1512:void[])
    n1000 = Divide(x=w1757, y=w1758) -> (x/y=w1756:dbl)
    "Buffer Status" <- w1756
    n1001 = To Unsigned Long Integer(number=w1511) -> (unsigned 32bit integer=w1510:u32[])
    n1002 = Join Numbers(hi=w1513, lo=w1512) -> ((hi.lo)=w1509:u32)
    n1003 = Equal?(x=w1756, y=1.0) -> (x = y?=w1754:bool)
    n1004 = Join Numbers(hi=w1510, lo=w1509) -> ((hi.lo)=w1503:u64[])
    n1005 = call "IR AOM word to freq - vec.vi"("Frequency Word In (double vec)"=w1503) -> ("Frequency Out"=w1550:dbl[])
    n1006 = case "Alert buffer overflow" shown="True" w1754 {
      frame False {
      }
      frame True {
        n1007 = call <vilib>:"Beep.vi"() -> ()  [unwired: 3 in, 9 out]
        "Overflow (data lost)" <- TRUE ("Overflow (data lost)")
      }
    }
    n1008 = Decimate 1D Array(w1550) -> (w1549:dbl[], w1548:dbl[])
    n1009 = Build Array(w1549, w1548) -> (w1547:dbl[][])
    n1010 = local read "Trap Sets"() -> (w1625:u32)
    n1011 = case "Deinterlace trap data, average down PSD" shown="2" w1625 {
      tunnel: w1515 -> [w2288 w2353]
      tunnel: [w2285 w2350] -> w1618
      tunnel: [w2288 w2352] -> w1506
      tunnel: "Detector Type" -> [w2287 w2348]
      tunnel: [w2286 w2351] -> w1617
      tunnel: [w2284 w2349] -> w1731
      frame 1, Default {
        n1012 = Divide(x=w2288, y=3276.7) -> (x/y=w2289:dbl)
        n1013 = Decimate 1D Array(w2289) -> (w2298:dbl[], w2297:dbl[], w2296:dbl[], w2295:dbl[], w2294:dbl[], w2293:dbl[], w2292:dbl[], w2291:dbl[])
        n1014 = case shown="\"IR-QPD + PSD + FB-QPD position\"" w2287 {
          tunnel: w2298 -> [w2322 w2347]
          tunnel: w2297 -> [w2321 w2346]
          tunnel: w2296 -> [w2306 w2324]
          tunnel: w2295 -> [w2307 w2334]
          tunnel: w2294 -> [w2320 w2345]
          tunnel: w2293 -> [w2319 w2344]
          tunnel: w2292 -> [w2303 w2325]
          tunnel: w2291 -> [w2302 w2323]
          tunnel: [w2301 w2331] -> w2286
          tunnel: [w2300 w2330] -> w2285
          tunnel: [w2299 w2329] -> w2284
          frame "IR-QPD + PSD + FB-QPD", Default {
            w2299 = 0  # Channel pattern
            n1015 = Divide(x=w2322, y=w2307) -> (x/y=w2309:dbl[])
            n1016 = Divide(x=w2321, y=w2307) -> (x/y=w2308:dbl[])
            n1017 = Divide(x=w2320, y=w2303) -> (x/y=w2305:dbl[])
            n1018 = Divide(x=w2319, y=w2302) -> (x/y=w2304:dbl[])
            n1019 = Build Array(w2309, w2308, w2307, w2306, w2305, w2304, w2303, w2302) -> (w2300:dbl[][])
            n1020 = Bundle("T1 Y", "T1 X", "T1 Sum", "FB Sum", "PSD Y", "PSD X", "PSD Y Sum", "PSD X Sum") -> (w2318:T37)  [unwired: 1 out]
            n1021 = Cluster To Array(cluster=w2318) -> (array=w2301:string[])
          }
          frame "IR-QPD + PSD + FB-QPD position" {
            w2329 = 3  # Channel pattern
            n1022 = Negate(x=w2325) -> (-x=w2326:dbl[])
            n1023 = Divide(x=w2347, y=w2334) -> (x/y=w2336:dbl[])
            n1024 = Divide(x=w2346, y=w2334) -> (x/y=w2335:dbl[])
            n1025 = Divide(x=w2345, y=w2325) -> (x/y=w2333:dbl[])
            n1026 = Divide(x=w2344, y=w2326) -> (x/y=w2332:dbl[])
            n1027 = Build Array(w2336, w2335, w2334, w2323, w2324, w2333, w2332, w2325) -> (w2330:dbl[][])
            n1028 = Bundle("T1 Y", "T1 X", "T1 Sum", "FB X", "FB Sum", "PSD Y", "PSD X", "PSD Y Sum") -> (w2343:T37)  [unwired: 1 out]
            n1029 = Cluster To Array(cluster=w2343) -> (array=w2331:string[])
          }
        }
      }
      frame 2 {
        n1030 = case shown="\"IR-QPD + PSD + FB-QPD X position\"" w2348 {
          tunnel: w2353 -> [w2415 w2482 w2553]
          tunnel: [w2354 w2473 w2484] -> w2352
          tunnel: [w2381 w2464 w2531] -> w2351
          tunnel: [w2380 w2427 w2498] -> w2350
          tunnel: [w2374 w2462 w2529] -> w2349
          frame "IR-QPD + PSD + FB-QPD", Default {
            w2374 = 1  # Channel pattern
            # "time average x2 the 4th signal and the 4 psd signals (detection laser)"
            # "deinterlace 3 signals from qpd"
            n1031 = Decimate 1D Array(w2415) -> (w2414:void[], w2413:void[], w2379:void[], w2412:void[], w2402:void[], w2400:void[], w2399:void[], w2397:void[])
            n1032 = Decimate 1D Array(w2379) -> (w2378:void[], w2377:void[])
            n1033 = Decimate 1D Array(w2414) -> (w2411:void[], w2383:void[])
            n1034 = Decimate 1D Array(w2413) -> (w2410:void[], w2408:void[])
            n1035 = Decimate 1D Array(w2412) -> (w2409:void[], w2407:void[])
            n1036 = call "downsample 1D array - double.vi"("Ave N"=2.0, "Array In"=w2402) -> ("Array Out"=w2401:dbl[])  [unwired: 1 out]
            n1037 = call "downsample 1D array - double.vi"("Ave N"=2.0, "Array In"=w2400) -> ("Array Out"=w2382:dbl[])  [unwired: 1 out]
            n1038 = call "downsample 1D array - double.vi"("Ave N"=2.0, "Array In"=w2399) -> ("Array Out"=w2398:dbl[])  [unwired: 1 out]
            n1039 = call "downsample 1D array - double.vi"("Ave N"=2.0, "Array In"=w2397) -> ("Array Out"=w2396:dbl[])  [unwired: 1 out]
            n1040 = Interleave 1D Arrays(w2411, w2410, w2409, w2383, w2408, w2407, w2378, w2377, w2401, w2382, w2398, w2396) -> (w2395:dbl[])
            n1041 = Divide(x=w2395, y=3276.7) -> (x/y=w2394:dbl[])
            n1042 = Decimate 1D Array(w2394) -> (w2393:dbl[], w2392:dbl[], w2391:dbl[], w2390:dbl[], w2389:dbl[], w2388:dbl[], w2376:dbl[], w2375:dbl[], w2387:dbl[], w2386:dbl[], w2385:dbl[], w2384:dbl[])
            n1043 = Divide(x=w2393, y=w2391) -> (x/y=w2361:dbl[])
            n1044 = Divide(x=w2392, y=w2391) -> (x/y=w2360:dbl[])
            n1045 = Divide(x=w2390, y=w2388) -> (x/y=w2359:dbl[])
            n1046 = Divide(x=w2389, y=w2388) -> (x/y=w2358:dbl[])
            n1047 = Divide(x=w2387, y=w2385) -> (x/y=w2357:dbl[])
            n1048 = Divide(x=w2386, y=w2384) -> (x/y=w2356:dbl[])
            n1049 = Build Array(w2361, w2360, w2391, w2359, w2358, w2388, w2376, w2375, w2357, w2356, w2385, w2384) -> (w2380:dbl[][])
            n1050 = Bundle("T1 Y", "T1 X", "T1 Sum", "T2 Y", "T2 X", "T2 Sum", "T1 FB Sum", "T2 FB Sum", "PSD Y", "PSD X", "PSD Y Sum", "PSD X Sum") -> (w2362:T38)  [unwired: 1 out]
            n1051 = To Word Integer(number=w2395) -> (16bit integer=w2354:i16[])
            n1052 = Cluster To Array(cluster=w2362) -> (array=w2381:string[])
          }
          frame "IR-QPD + PSD + FB-QPD X position" {
            w2462 = 2  # Channel pattern
            # "time average x2 the 3 psd signals (detection laser)"
            # "deinterlace 3 signals from qpds"
            n1053 = Decimate 1D Array(w2482) -> (w2481:void[], w2480:void[], w2463:void[], w2479:void[], w2425:void[], w2422:void[], w2419:void[], w2450:void[])
            n1054 = Decimate 1D Array(w2463) -> (w2448:void[], w2446:void[])
            n1055 = Decimate 1D Array(w2481) -> (w2478:void[], w2465:void[])
            n1056 = Decimate 1D Array(w2480) -> (w2477:void[], w2475:void[])
            n1057 = Decimate 1D Array(w2479) -> (w2476:void[], w2474:void[])
            n1058 = Decimate 1D Array(w2450) -> (w2449:void[], w2447:void[])
            n1059 = call "downsample 1D array - I16.vi"("Ave N"=2.0, "Array In"=w2425) -> ("Array Out"=w2423:i16[])  [unwired: 1 in]
            n1060 = call "downsample 1D array - I16.vi"("Ave N"=2.0, "Array In"=w2419) -> ("Array Out"=w2417:i16[])  [unwired: 1 in]
            n1061 = call "downsample 1D array - I16.vi"("Ave N"=2.0, "Array In"=w2422) -> ("Array Out"=w2420:i16[])  [unwired: 1 in]
            n1062 = Interleave 1D Arrays(w2478, w2477, w2476, w2465, w2475, w2474, w2449, w2448, w2447, w2446, w2423, w2420, w2417) -> (w2473:i16[])
            n1063 = Divide(x=w2473, y=3276.7) -> (x/y=w2472:dbl[])
            n1064 = Decimate 1D Array(w2472) -> (w2471:dbl[], w2470:dbl[], w2469:dbl[], w2468:dbl[], w2467:dbl[], w2466:dbl[], w2438:dbl[], w2436:dbl[], w2435:dbl[], w2433:dbl[], w2432:dbl[], w2431:dbl[], w2428:dbl[])
            n1065 = Negate(x=w2428) -> (-x=w2426:dbl[])
            n1066 = Divide(x=w2432, y=w2428) -> (x/y=w2430:dbl[])
            n1067 = Divide(x=w2431, y=w2426) -> (x/y=w2429:dbl[])
            n1068 = Divide(x=w2471, y=w2469) -> (x/y=w2454:dbl[])
            n1069 = Divide(x=w2470, y=w2469) -> (x/y=w2453:dbl[])
            n1070 = Divide(x=w2468, y=w2466) -> (x/y=w2452:dbl[])
            n1071 = Divide(x=w2467, y=w2466) -> (x/y=w2451:dbl[])
            n1072 = Divide(x=w2438, y=w2436) -> (x/y=w2437:dbl[])
            n1073 = Divide(x=w2435, y=w2433) -> (x/y=w2434:dbl[])
            n1074 = Build Array(w2454, w2453, w2469, w2452, w2451, w2466, w2437, w2436, w2434, w2433, w2430, w2429, w2428) -> (w2427:dbl[][])
            n1075 = Bundle("T1 Y", "T1 X", "T1 Sum", "T2 Y", "T2 X", "T2 Sum", "T1 FB X", "T1 FB Sum", "T2 FB X", "T2 FB Sum", "PSD Y", "PSD X", "PSD Y Sum") -> (w2455:T39)  [unwired: 1 out]
            n1076 = Cluster To Array(cluster=w2455) -> (array=w2464:string[])
          }
          frame "IR-QPD + PSD + FB-QPD XY positions" {
            w2529 = 4  # Channel pattern
            # "time average x2 the 3 psd signals (detection laser)"
            # "deinterlace 3 signals from qpds"
            n1077 = Decimate 1D Array(w2553) -> (w2552:void[], w2551:void[], w2530:void[], w2550:void[], w2496:void[], w2542:void[], w2541:void[], w2518:void[])
            n1078 = Decimate 1D Array "Feedback Sum"(w2530) -> (w2514:void[], w2512:void[])
            n1079 = Decimate 1D Array "QPD Y"(w2552) -> (w2549:void[], w2532:void[])
            n1080 = Decimate 1D Array "QPD X"(w2551) -> (w2548:void[], w2546:void[])
            n1081 = Decimate 1D Array "Feedback Y"(w2496) -> (w2495:void[], w2494:void[])
            n1082 = Decimate 1D Array "QPD Sum"(w2550) -> (w2547:void[], w2545:void[])
            n1083 = Decimate 1D Array "Feedback X"(w2518) -> (w2515:void[], w2513:void[])
            n1084 = call "downsample 1D array - double.vi"("Ave N"=2.0, "Array In"=w2542) -> ("Array Out"=w2517:dbl[])  [unwired: 1 out]
            n1085 = call "downsample 1D array - double.vi"("Ave N"=2.0, "Array In"=w2541) -> ("Array Out"=w2516:dbl[])  [unwired: 1 out]
            n1086 = Interleave 1D Arrays(w2549, w2548, w2547, w2532, w2546, w2545, w2495, w2515, w2514, w2494, w2513, w2512, w2517, w2516) -> (w2540:dbl[])
            n1087 = Divide(x=w2540, y=3276.7) -> (x/y=w2539:dbl[])
            n1088 = Decimate 1D Array(w2539) -> (w2538:dbl[], w2537:dbl[], w2536:dbl[], w2535:dbl[], w2534:dbl[], w2533:dbl[], w2491:dbl[], w2505:dbl[], w2489:dbl[], w2490:dbl[], w2503:dbl[], w2487:dbl[], w2501:dbl[], w2499:dbl[])
            n1089 = Negate(x=w2499) -> (-x=w2497:dbl[])
            n1090 = Divide(x=w2501, y=w2497) -> (x/y=w2500:dbl[])
            n1091 = Divide(x=w2490, y=w2487) -> (x/y=w2486:dbl[])
            n1092 = Divide(x=w2491, y=w2489) -> (x/y=w2488:dbl[])
            n1093 = Divide(x=w2538, y=w2536) -> (x/y=w2522:dbl[])
            n1094 = Divide(x=w2537, y=w2536) -> (x/y=w2521:dbl[])
            n1095 = Divide(x=w2535, y=w2533) -> (x/y=w2520:dbl[])
            n1096 = Divide(x=w2534, y=w2533) -> (x/y=w2519:dbl[])
            n1097 = Divide(x=w2505, y=w2489) -> (x/y=w2504:dbl[])
